vi "String To AP Sx Bits.vi"(8 "error in (no error)":errorcluster caption="错误输入（无错误）", 9 "autoDetectAsicType":i32, 10 "bitsBuffer":string, 11 "asicHandle":i32) -> (0 "error out":errorcluster caption="错误输出", 2 "bitsBuffer out":string, 3 "function return":i32)   [LabVIEW 2018]
doc: "extern int __stdcall StringToAPSxBits (int asicHandle, IN char bitsBuffer[], IN int autoDetectAsicType);"
uses:
  APSx.dll/APSx.dll
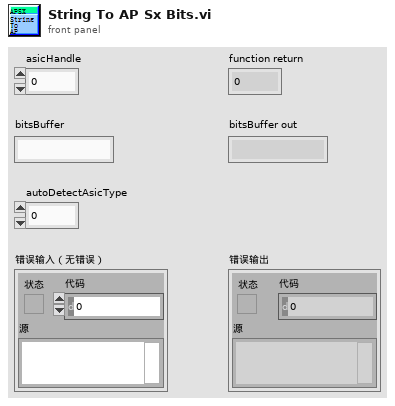
[diagram p1: front panel]
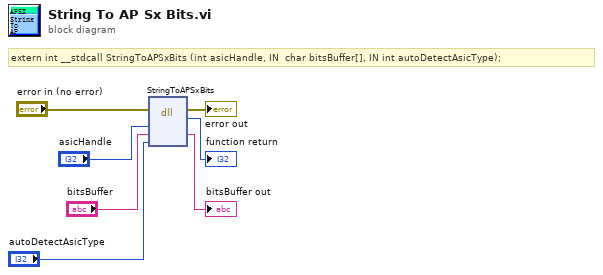
[diagram p0: block diagram]
diagram:
  # "extern int __stdcall StringToAPSxBits (int asicHandle, IN  char bitsBuffer[], IN int autoDetectAsicType);"
  n1 = dll-call lib="PTH2[abs D项目Feng恒隆项目Labview传感器对中台SourcesAPSx.dllAPSx.*" fn="StringToAPSxBits"(error in="error in (no error)", "asicHandle"="asicHandle", "bitsBuffer"="bitsBuffer", "autoDetectAsicType"="autoDetectAsicType") -> (error out=→"error out":errorcluster, →"function return":i32, "bitsBuffer"=→"bitsBuffer out":string)  [unwired: 4 in, 1 out]
